vi "NMAK_SubVI.vi"(10 "min time SCL High (uSEC)":u32 caption="Count(min time SCL High (uSEC))", 11 "min time SCL Low (uSEC)":u32) -> ()   [LabVIEW 2019]
uses:
  <vilib>/rvi/eio/common/nirviEmuTemplateMethod_errors.vi
  <vilib>/eio/EIONode/EIONode.xnode
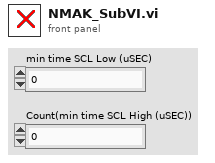
[diagram p1: front panel]
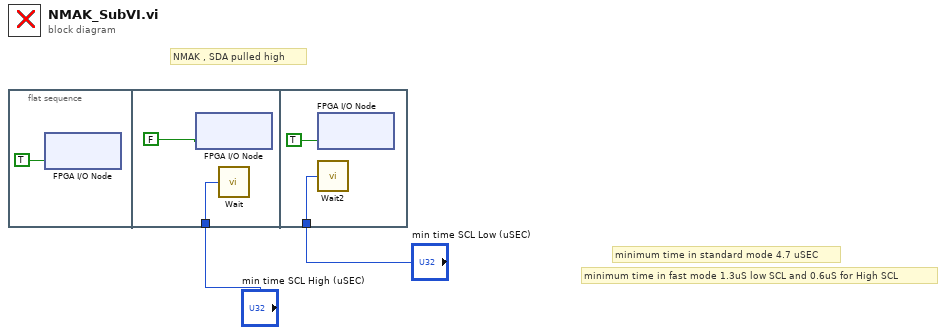
[diagram p0: block diagram]
diagram:
  # "NMAK , SDA pulled high"
  # "minimum time in fast mode 1.3uS low SCL and 0.6uS for High SCL"
  # "minimum time in standard mode 4.7 uSEC"
  n1 = flat-sequence {
    tunnel: "min time SCL High (uSEC)" -> [w5]
    tunnel: "min time SCL Low (uSEC)" -> [w7]
    frame #0 {
      n2 = xnode "FPGA I/O Node"("SDA"=TRUE) -> ()  [unwired: 1 in, 1 out]
    }
    frame #1 {
      n3 = xnode "FPGA I/O Node"("SCL"=FALSE) -> ()  [unwired: 1 in, 1 out]
      n4 = call "Wait"("Count(Ticks)"=w5) -> ()  [unwired: 1 out]
    }
    frame #2 {
      n5 = xnode "FPGA I/O Node"("SCL"=TRUE) -> ()  [unwired: 1 in, 1 out]
      n6 = call "Wait2"("Count(Ticks)"=w7) -> ()  [unwired: 1 out]
    }
  }
